vi "query_command_packet.vi"(8 "error in (no error)":errorcluster, 10 "command packet":string, 11 "VISA resource name":refnum<visa-resource-name>) -> (0 "error out":errorcluster, 1 "response packet cluster":T1, 2 "response":string, 3 "VISA resource name out":refnum<visa-resource-name>)   [LabVIEW 2018]
doc: "Write a command packet to the IC6 and read the response packet, checking for errors in the query cycle.\n\nThis VI will only read the response packet correctly if there is a single command in the message portion of the command packet. This is a limitation imposed by this driver library, not the instrument."
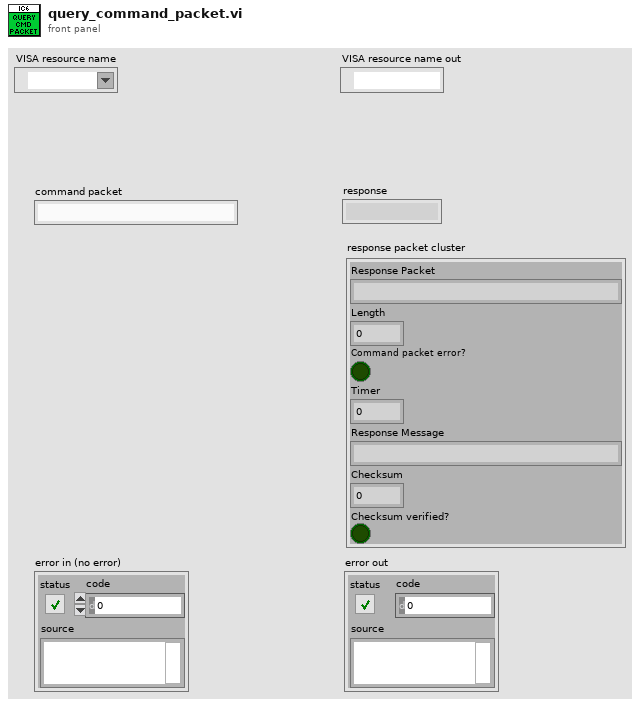
[diagram p1: front panel]
types:
  T1 = cluster{"Response Packet":string, "Length":u16, "Command packet error?":bool, "Timer":u8, "Response Message":string, "Checksum":u8, "Checksum verified?":bool}
  T2 = enum16{"big-endian, network order", "native, host order", "little-endian"}
  T3 = enum16{"Command packet error", "Checksum not verified", "Command not acknowledged"}
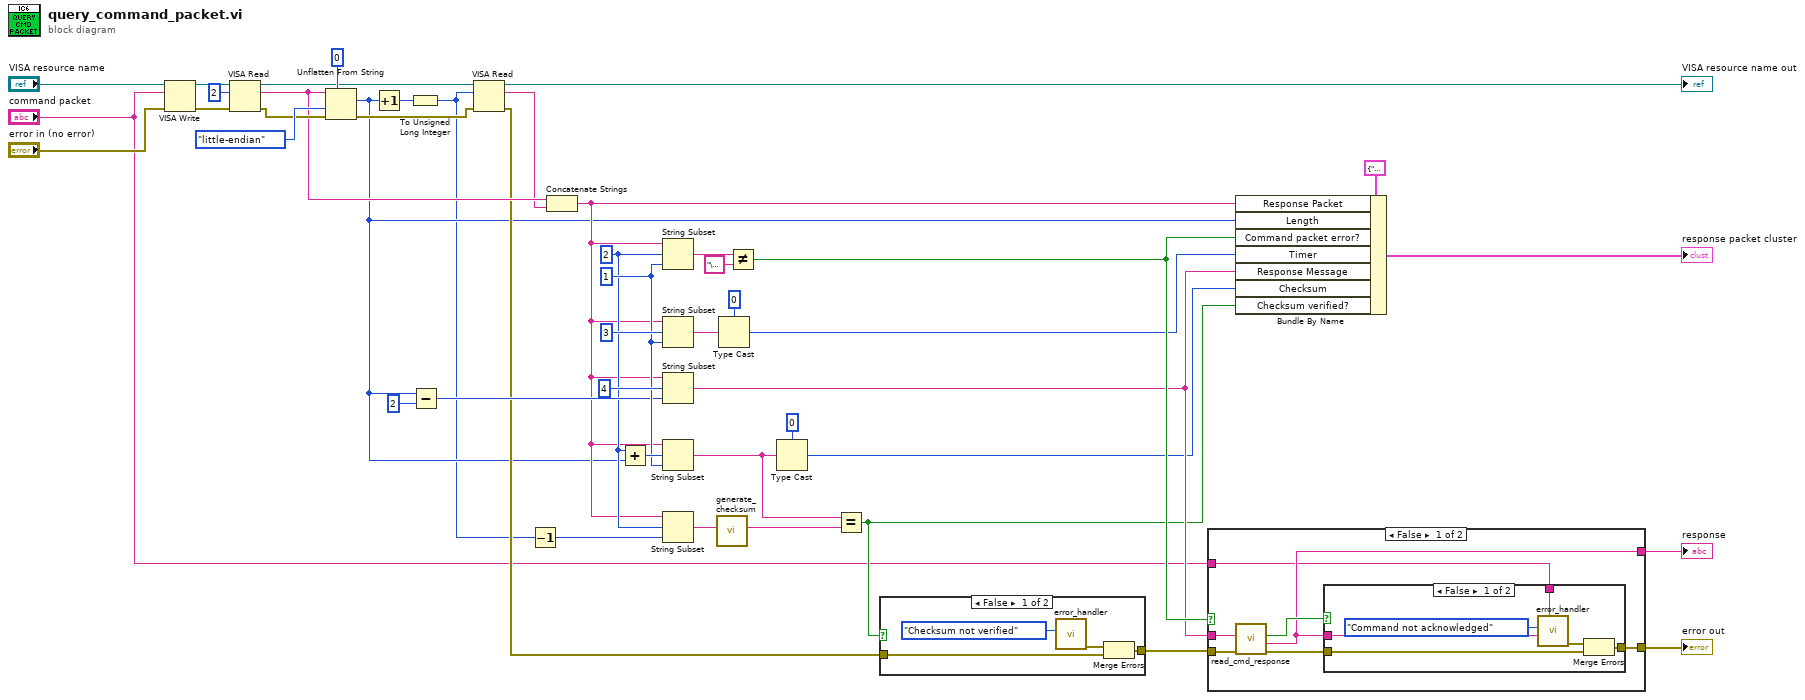
[diagram p0: block diagram]
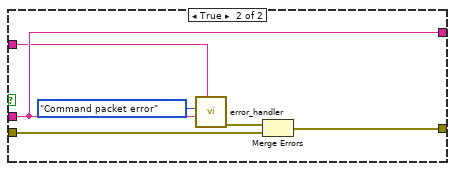
[diagram p4: hidden frame]
diagram:
  w33 = 1 ("length (rest)")
  w18 = 2 ("offset (0)")
  n1 = VISA Write(VISA resource name="VISA resource name", write buffer="command packet", error in (no error)="error in (no error)") -> (VISA resource name out=w45:refnum<visa-resource-name>, error out=w39:errorcluster)  [unwired: 1 out]
  n2 = VISA Read(VISA resource name=w45, byte count=u32 2 ("bytes to read"), error in (no error)=w39) -> (VISA resource name out=w6:refnum<visa-resource-name>, read buffer=w32:string, error out=w38:errorcluster)  [unwired: 1 out]
  n3 = Unflatten From String(type=u16 0, binary string=w32, byte order (0:big-endian, network order)=T2."little-endian", error in (no error)=w38) -> (value=w4:u16, error out=w37:errorcluster)  [unwired: 1 in, 1 out]
  n4 = Increment(x=w4) -> (x+1=w41:u16)
  n5 = To Unsigned Long Integer(number=w41) -> (unsigned 32bit integer=w2:u32)
  n6 = Subtract(x=w4, y=u16 2) -> (x-y=w23:u16)
  n7 = VISA Read(VISA resource name=w6, byte count=w2, error in (no error)=w37) -> (VISA resource name out=→"VISA resource name out":refnum<visa-resource-name>, read buffer=w26:string, error out=w17:errorcluster)  [unwired: 1 out]
  n8 = Decrement(x=w2) -> (x-1=w3:u32)
  n9 = Concatenate Strings(w32, w26) -> (w11:string)
  n10 = Add(x=w18, y=w4) -> (x+y=w34:i32)
  n11 = String Subset(string=w11, offset (0)=w18, length (rest)=w33) -> (substring=w30:string)
  n12 = String Subset(string=w11, offset (0)=3, length (rest)=w33) -> (substring=w28:string)
  n13 = String Subset(string=w11, offset (0)=4, length (rest)=w23) -> (substring=w12:string)
  n14 = String Subset(string=w11, offset (0)=w34, length (rest)=w33) -> (substring=w21:string)
  n15 = String Subset(string=w11, offset (0)=w18, length (rest)=w3) -> (substring=w25:string)
  n16 = call "generate_checksum.vi"("message"=w25) -> ("checksum"=w22:string)  [unwired: 10 in]
  n17 = Type Cast(type=u8 0 ("value"), x=w28) -> (*(type *) &x=w10:u8)
  n18 = Not Equal?(x=w30, y="\u0000") -> (x != y?=w13:bool)
  n19 = Type Cast(type=u8 0 ("value"), x=w21) -> (*(type *) &x=w9:u8)
  n20 = Equal?(x=w21, y=w22) -> (x = y?=w8:bool)
  n21 = case shown="False" w8 {
    tunnel: w17 -> [w48 w50]
    tunnel: [w47 w50] -> w16
    frame False {
      n22 = call "error_handler.vi"("Error type"=T3."Checksum not verified") -> ("error out"=w49:errorcluster)  [unwired: 10 in]
      n23 = Merge Errors(w49, w48) -> (w47:errorcluster)
    }
    frame True {
    }
  }
  n24 = case shown="False" w13 {
    tunnel: w16 -> [w54 w69]
    tunnel: [w55 w68] -> w15
    tunnel: w12 -> [w56 w66]
    tunnel: [w52 w66] -> w14
    tunnel: "command packet" -> [w51 w65]
    frame False {
      n25 = call "read_cmd_response.vi"("error in (no error)"=w54, "command response"=w56) -> ("error out"=w53:errorcluster, "response"=w52:string, "acknowledged?"=w57:bool)  [unwired: 7 in]
      n26 = case shown="False" w57 {
        tunnel: w53 -> [w62 w64]
        tunnel: [w61 w64] -> w55
        tunnel: w52 -> [w60 _]
        tunnel: w51 -> [w58 _]
        frame False {
          n27 = call "error_handler.vi"("command"=w58, "IC6 error code"=w60, "Error type"=T3."Command not acknowledged") -> ("error out"=w63:errorcluster)  [unwired: 8 in]
          n28 = Merge Errors(w63, w62) -> (w61:errorcluster)
        }
        frame True {
        }
      }
    }
    frame True {
      n29 = call "error_handler.vi"("command"=w65, "IC6 error code"=w66, "Error type"=T3."Command packet error") -> ("error out"=w70:errorcluster)  [unwired: 8 in]
      n30 = Merge Errors(w70, w69) -> (w68:errorcluster)
    }
  }
  "error out" <- w15
  "response" <- w14
  n31 = Bundle By Name(cluster=T1 {"Response Packet"="", "Length"=0, "Command packet error?"=FALSE, "Timer"=0, "Response Message"="", "Checksum"=0, "Checksum verified?"=FALSE} ("Response packet cluster"), "Response Packet"=w11, "Length"=w4, "Command packet error?"=w13, "Timer"=w10, "Response Message"=w12, "Checksum"=w9, "Checksum verified?"=w8) -> (→"response packet cluster":T1)
